vi "max_regelung.vi"(5 "TI 21a IW °C":dbl, 6 "Drehzahl IW u/min":dbl, 8 "delta P IW bar":dbl, 9 "FI 13 IW l/min":dbl, 10 "FI 13 SW l/min":dbl(slide)=3.0 min=3.0 max=12.0 step=0.1 scale=3.0..12.0, 11 "TI 02 IW °C":dbl) -> (0 "y u/min":dbl, 1 "y V":dbl, 2 "zu":bool=TRUE, 3 "auf":bool=TRUE)   [LabVIEW 2015]
panel:
  in  "PT1 Faktor":dbl=2.0000000000000004
  in  "PT1 Tau":dbl=10.0
  in  "TI 21a SW °C":dbl=60.0 min=30.0 max=60.0
  in  "i":dbl format="%#_13g"
  in  "Haltezeit s":dbl=4.0 min=0.0 max=15.0 step=1.0
  in  "Pumpe":bool
  in  "SP2":dbl=-0.15
  in  "SP4":dbl=0.2
  in  "SP1":dbl=-0.2
  in  "SP3":dbl=0.15
  in  "Öl-Regelung":bool
  # "Regelparameter"
  # "Regelparameter"
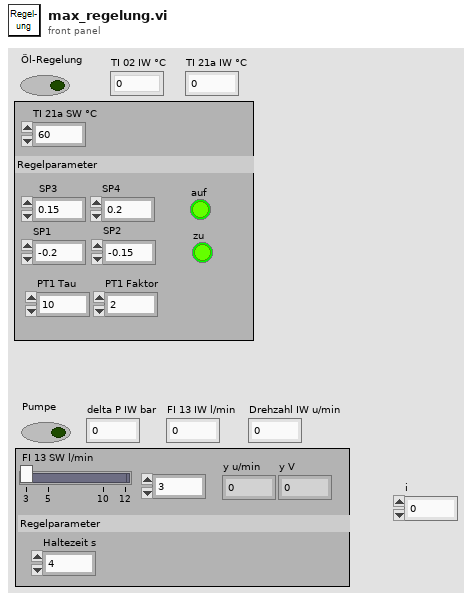
[diagram p1: front panel]
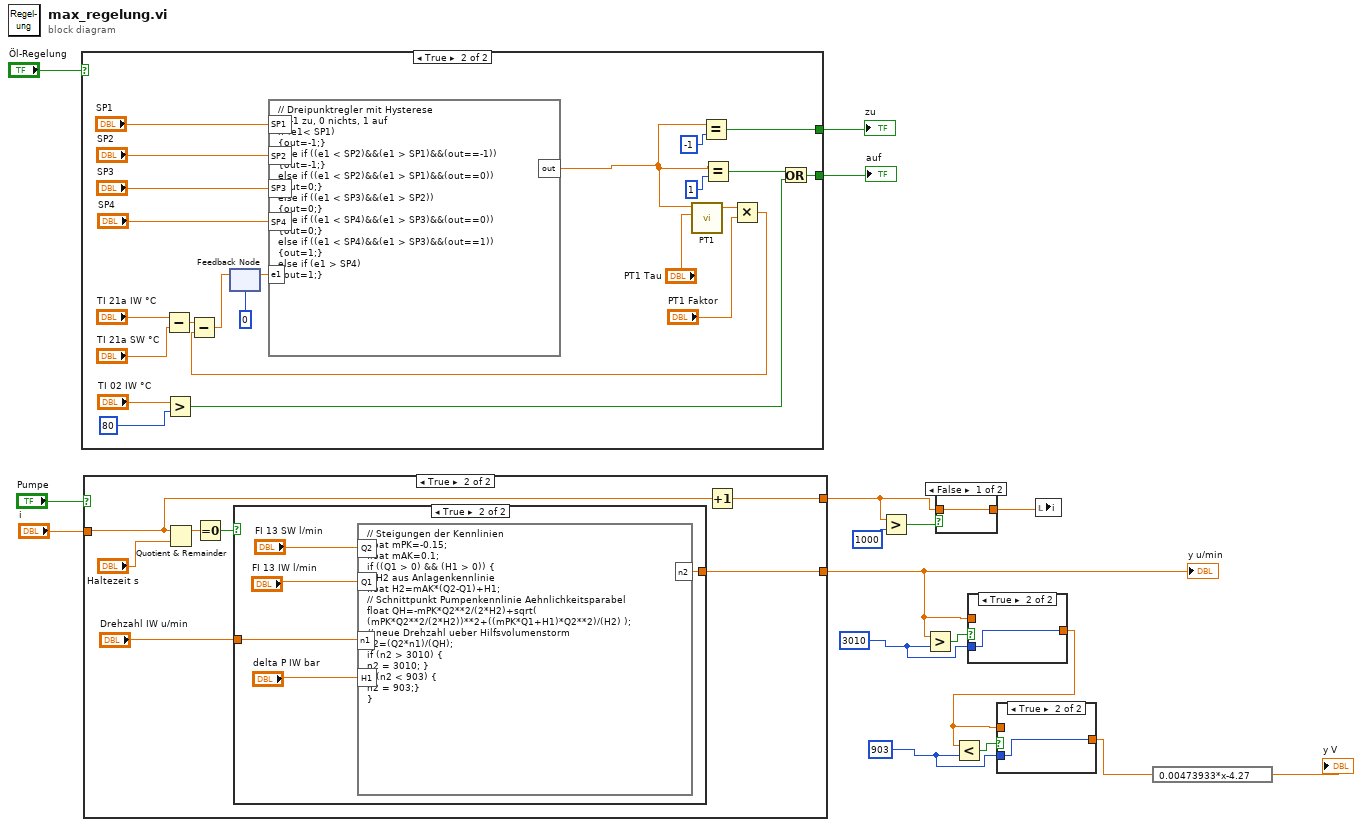
[diagram p0: block diagram]
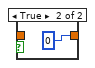
[diagram p4: hidden frame]
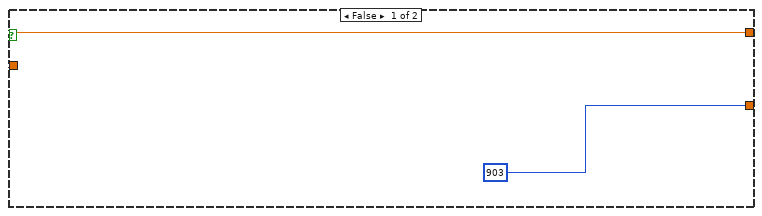
[diagram p5: hidden frame]
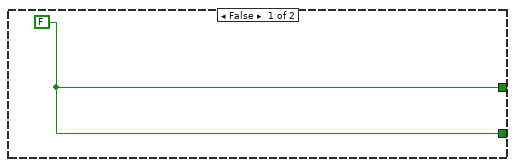
[diagram p7: hidden frame]
diagram:
  w3 = 903
  w5 = 3010
  n1 = case shown="True" "Öl-Regelung" {
    tunnel: [w18 w37] -> w16
    tunnel: [w18 w23] -> w15
    frame False {
      w18 = FALSE
    }
    frame True {
      n2 = Subtract(x="TI 21a IW °C", y="TI 21a SW °C") -> (x-y=w31:dbl)
      n3 = Greater?(x="TI 02 IW °C", y=80) -> (0:w22:bool)
      n4 = feedback #1(0) -> (w28:dbl)
      n5 = formula code="// Dreipunktregler mit Hysterese\n//  -1 zu, 0 nichts, 1 auf\nif (e1< SP1)\n{out=-1;}\nelse if ((e1 < SP2)&&(e1 > SP1)&&(out==-1))\n{out=-1;}\nelse if ((e1 < SP2)&&(e1 > SP1)&&(out==0))\n{out=0;}\nelse if ((e1 < SP3)&&(e1 > SP2))\n{out=0;}\nelse if ((e1 < SP4)&&(e1 > SP3)&&(out==0))\n{out=0;}\nelse if ((e1 < SP4)&&(e1 > SP3)&&(out==1))\n{out=1;}\nelse if (e1 > SP4)\n{out=1;}"("e1"=w28, "SP1"="SP1", "SP3"="SP3", "SP4"="SP4", "SP2"="SP2") -> ("out"=w19:dbl)
      n6 = call "PT1.vi"("Zeitkonstante(Tau)"="PT1 Tau", "Eingang"=w19) -> ("Ausgang"=w21:dbl)  [unwired: 9 in]
      n7 = Equal?(x=w19, y=-1) -> (x = y?=w37:bool)
      n8 = Equal?(x=w19, y=1) -> (x = y?=w24:bool)
      n9 = Multiply(x=w21, y="PT1 Faktor") -> (x*y=w30:dbl)
      n10 = Subtract(x=w31, y=w30) -> (x-y=w29:dbl)
      n11 = feedback-in #1(w29) -> ()
      n12 = Or(x=w24, y=w22) -> (x .or. y?=w23:bool)
    }
  }
  "zu" <- w16
  "auf" <- w15
  n13 = case shown="True" "Pumpe" {
    tunnel: [903 w44] -> w6
    tunnel: "i" -> [w42 w47]
    tunnel: [w42 w46] -> w11
    frame False {
    }
    frame True {
      n14 = Quotient & Remainder(x=w47, y="Haltezeit s") -> (x-y*floor(x/y)=w49:dbl)  [unwired: 1 out]
      n15 = Equal To 0?(x=w49) -> (x = 0?=w48:bool)
      n16 = case shown="True" w48 {
        tunnel: [w51 w54] -> w44
        tunnel: "Drehzahl IW u/min" -> [w51 w53]
        frame False {
        }
        frame True {
          n17 = formula code="// Steigungen der Kennlinien\nfloat mPK=-0.15;\nfloat mAK=0.1;\nif ((Q1 > 0) && (H1 > 0)) {\n// H2 aus Anlagenkennlinie\nfloat H2=mAK*(Q2-Q1)+H1;\n// Schnittpunkt Pumpenkennlinie Aehnlichkeitsparabel\nfloat QH=-mPK*Q2**2/(2*H2)+sqrt(\n(mPK*Q2**2/(2*H2))**2+((mPK*Q1+H1)*Q2**2)/(H2) );\n// neue Drehzahl ueber Hilfsvolumenstorm\nn2=(Q2*n1)/(QH);\nif (n2 > 3010) {\nn2 = 3010; }\nif (n2 < 903) {\nn2 = 903;}\n}"("Q1"="FI 13 IW l/min", "Q2"="FI 13 SW l/min", "n1"=w53, "H1"="delta P IW bar") -> ("n2"=w54:dbl)
        }
      }
      n18 = Increment(x=w47) -> (x+1=w46:dbl)
    }
  }
  "y u/min" <- w6
  n19 = Greater?(x=w11, y=1000) -> (0:w12:bool)
  n20 = Greater?(x=w6, y=w5) -> (0:w7:bool)
  n21 = case shown="False" w12 {
    tunnel: [w57 0] -> w9
    tunnel: w11 -> [w57 _]
    frame False {
    }
    frame True {
    }
  }
  n22 = case shown="True" w7 {
    tunnel: w6 -> [w59 _]
    tunnel: w5 -> [_ w60]
    tunnel: [w59 w60] -> w2
    frame False {
    }
    frame True {
    }
  }
  n23 = Less?(x=w2, y=w3) -> (x < y?=w4:bool)
  n24 = case shown="True" w4 {
    tunnel: w2 -> [w61 _]
    tunnel: w3 -> [_ w62]
    tunnel: [w61 w62] -> w1
    frame False {
    }
    frame True {
    }
  }
  n25 = local write "i"(w9) -> ()
  n26 = expression code="0.00473933*x-4.27"(w1) -> (→"y V":dbl)
